vi "ocw.vi"(1 "in":string) -> ()   [LabVIEW 2010]
doc: "OCW v3.0\n\nCopyright 2008 by Will Grover\n\nhttp://wgrover.com\n\nPermission is hereby granted, free of charge, to any person obtaining a copy of this software and associated documentation files (the \"Software\"), to deal in the Software without restriction, including without limitation the rights to use, copy, modify, merge, publish, distribute, sublicense, and/or sell copies of the Software, and to permit persons to whom the Software is furnished to do so, subject to the following conditions:\n\nThe above copyright notice and this permission notice shall be included in all copies or substantial portions of the Software.\n\nTHE SOFTWARE IS PROVIDED \"AS IS\", WITHOUT WARRANTY OF ANY KIND, EXPRESS OR IMPLIED, INCLUDING BUT NOT LIMITED TO THE WARRANTIES OF MERCHANTABILITY, FITNESS FOR A PARTICULAR PURPOSE AND NONINFRINGEMENT. IN NO EVENT SHALL THE AUTHORS OR COPYRIGHT HOLDERS BE LIABLE FOR ANY CLAIM, DAMAGES OR OTHER LIABILITY, WHETHER IN AN ACTION OF CONTRACT, TORT OR OTHERWISE, ARISING FROM, OUT OF OR IN CONNECTION WITH THE SOFTWARE OR THE USE OR OTHER DEALINGS IN THE SOFTWARE."
uses:
  Instance           1 11Saved   ocw .vi
panel:
  out "Subfunction stack":string[](array[string])=["pumpright", "main"]
  in  "Escape":bool
  out "Messages":string
  # "Make sure listener.vi is running before running this VI."
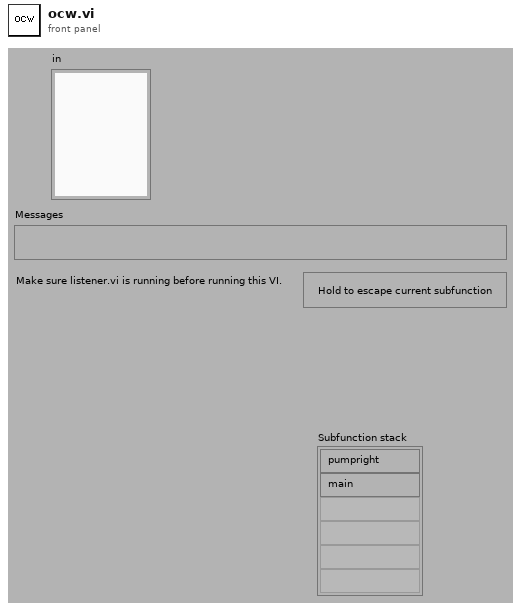
[diagram p1: front panel]
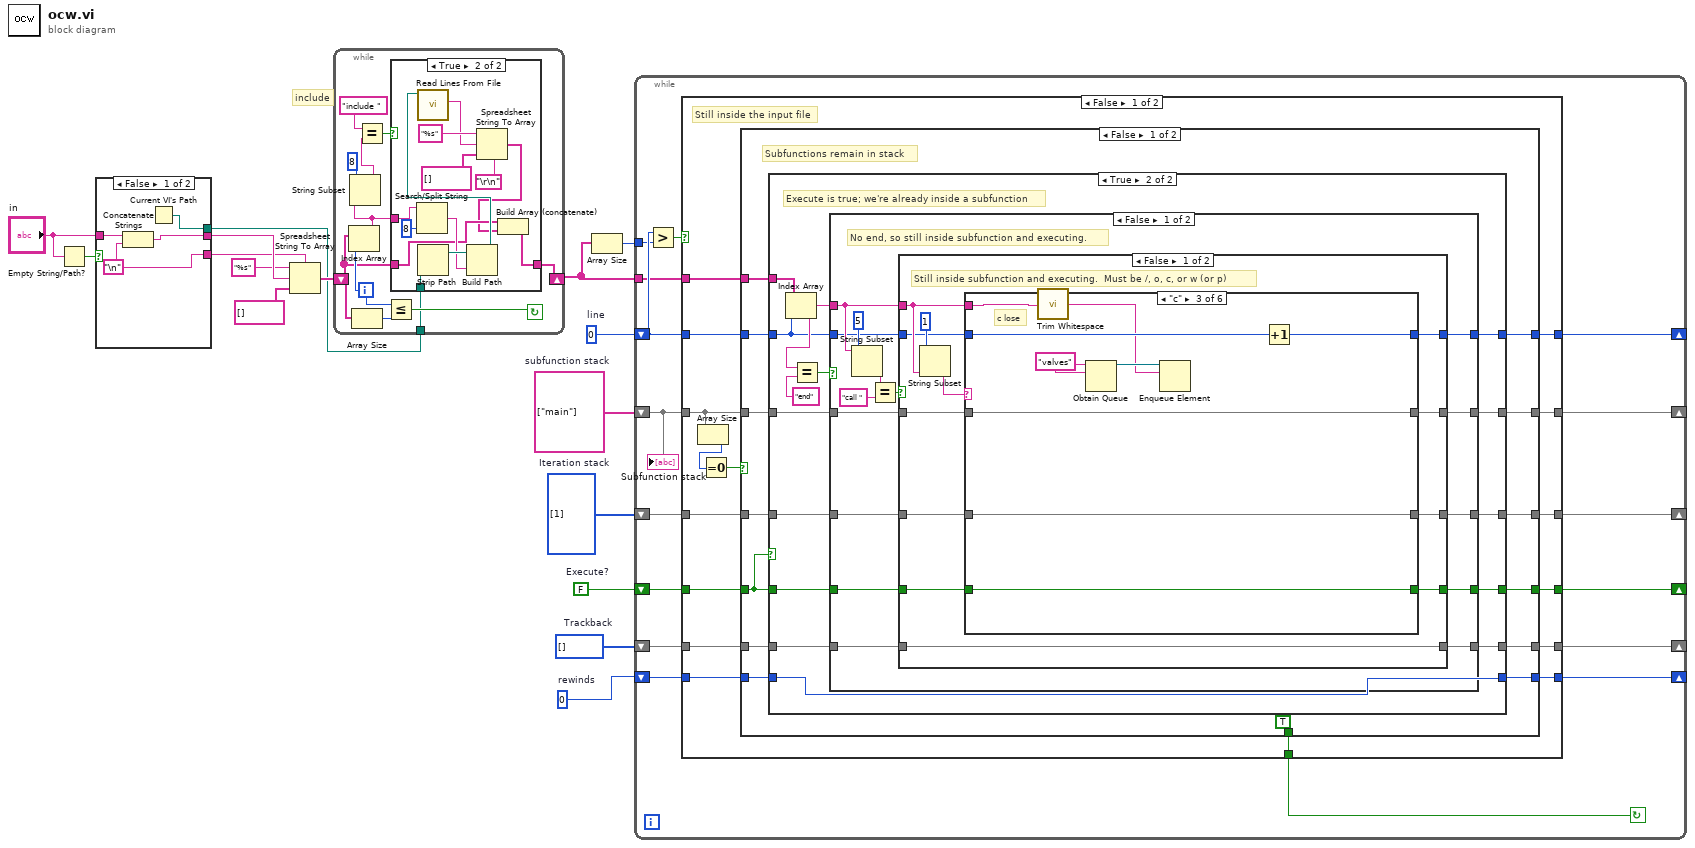
[diagram p0: block diagram]
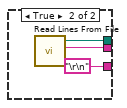
[diagram p2: hidden frame]
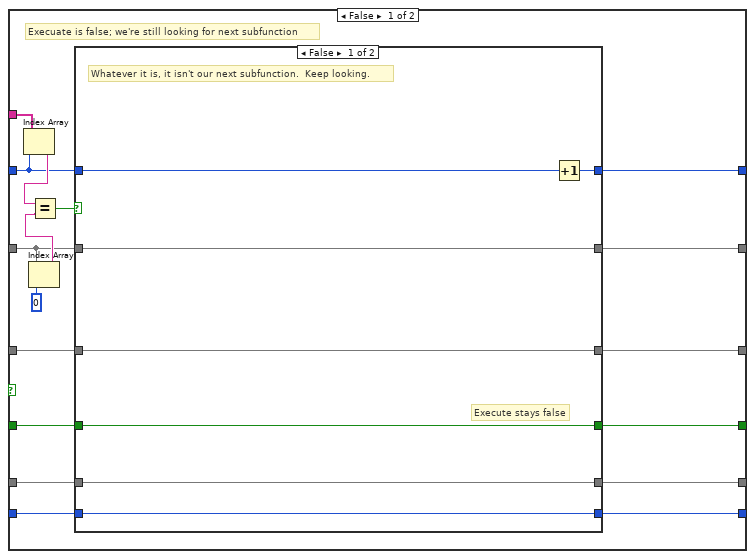
[diagram p4: hidden frame]
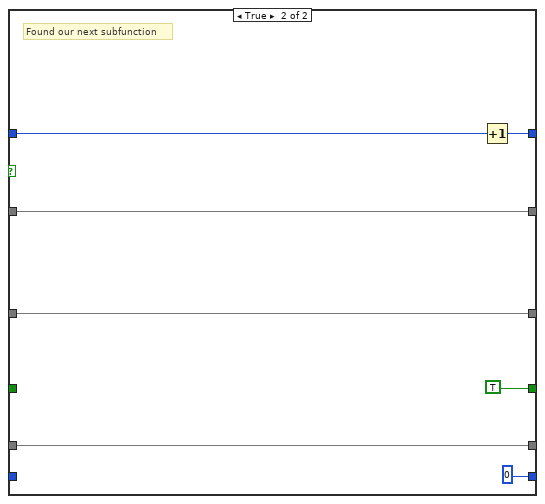
[diagram p5: hidden frame]
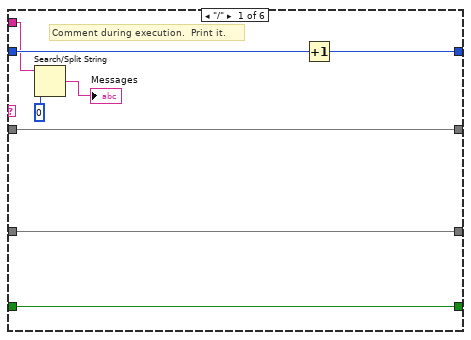
[diagram p6: hidden frame]
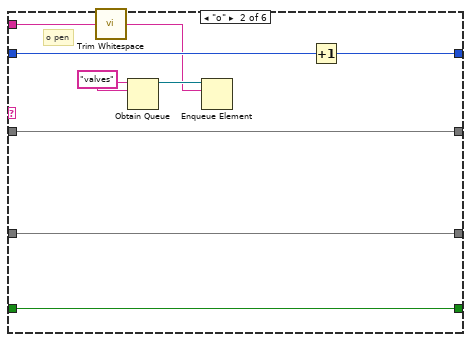
[diagram p7: hidden frame]
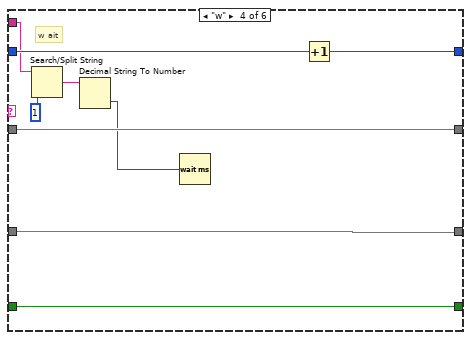
[diagram p8: hidden frame]
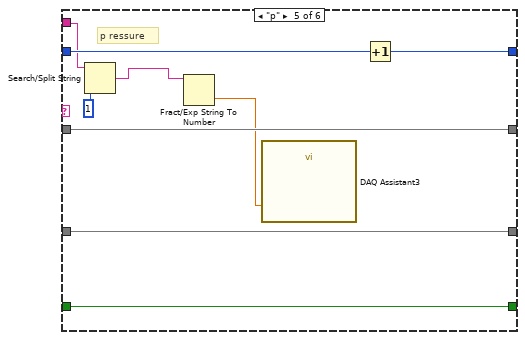
[diagram p9: hidden frame]
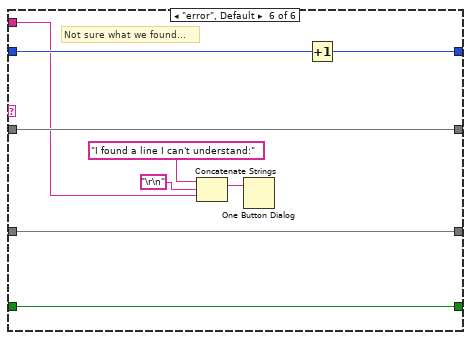
[diagram p10: hidden frame]
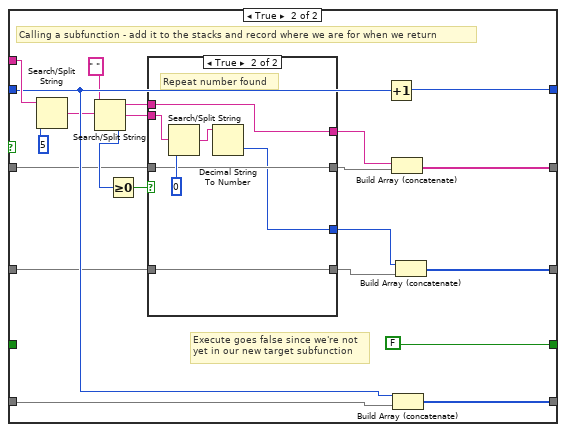
[diagram p11: hidden frame]
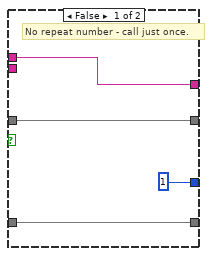
[diagram p12: hidden frame]
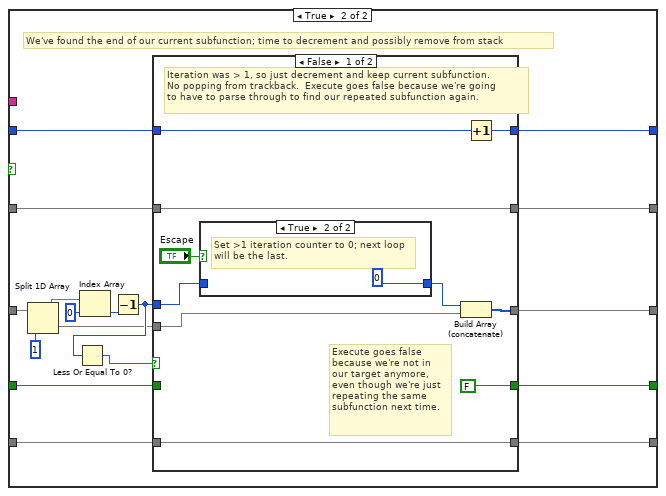
[diagram p13: hidden frame]
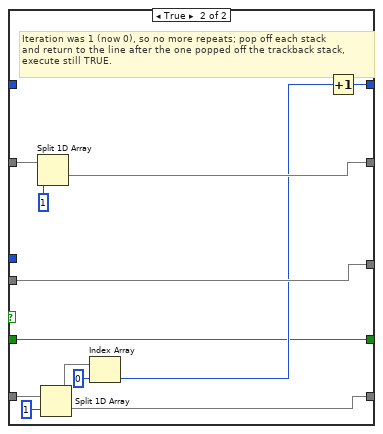
[diagram p15: hidden frame]
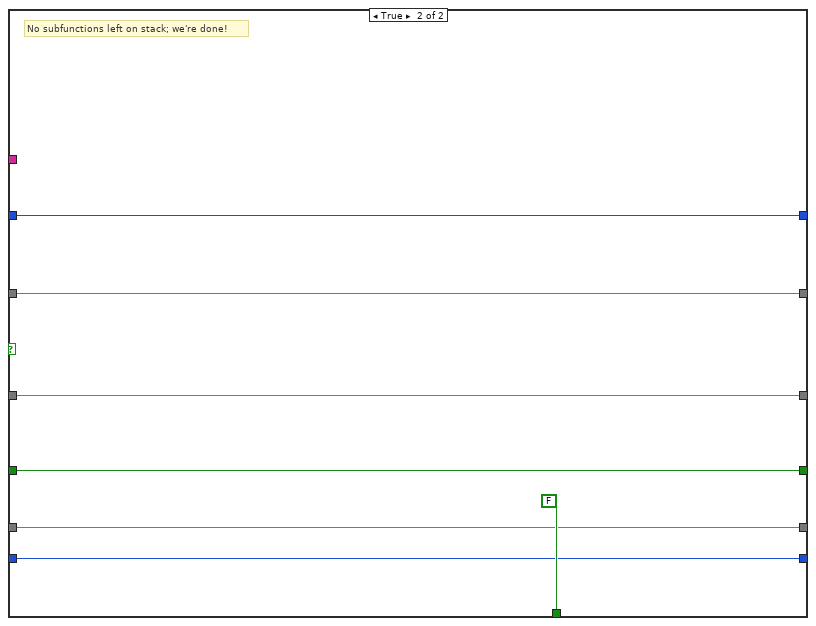
[diagram p16: hidden frame]
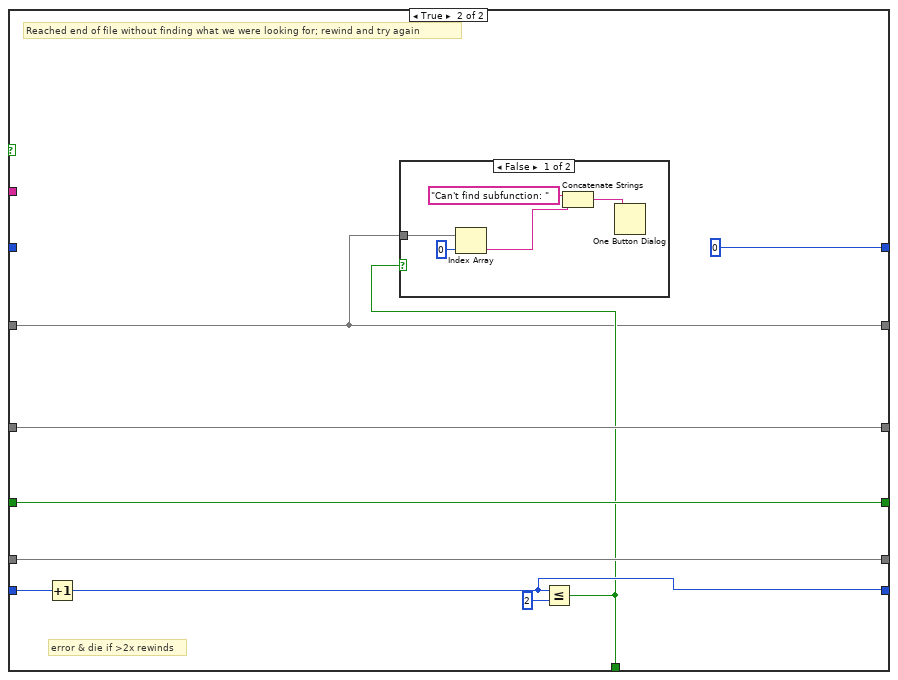
[diagram p17: hidden frame]
diagram:
  w9 = 0  # rewinds
  w11 = i32[] []  # Trackback
  w13 = 0  # line
  w14 = FALSE  # Execute?
  w15 = i32[] [1]  # Iteration stack
  w16 = string[] ["main"]  # subfunction stack
  # "include"
  n1 = Empty String/Path?(string/path="in") -> (empty?=w2:bool)
  n2 = case shown="False" w2 {
    tunnel: [w17 w23] -> w8
    tunnel: [w20 w22] -> w4
    tunnel: "in" -> [w19 _]
    tunnel: [w18 "\r\n"] -> w1
    frame False {
      w18 = "\n"
      n3 = Concatenate Strings(w19, w18) -> (w17:string)
      n4 = Current VI's Path() -> (path=w20:path)
    }
    frame True {
      n5 = call <vilib>:"Read Lines From File.vi"() -> ("new file path (Not A Path if cancelled)"=w22:path, "line string"=w23:string)  [unwired: 2 in, 6 out]
    }
  }
  n6 = Spreadsheet String To Array(delimiter (Tab)=w1, format string="%s", spreadsheet string=w8, array type (2D Dbl)=string[] [] ("Array Constant")) -> (array=w5:string[])
  n7 = while {
    tunnel: w4 -> [w24]
    shift-left: w5 -> [w26]
    shift-right: [w25] -> w10
    i -> [w34]
    stop <- w32 continue-if-true
    n8 = Index Array(array=w26, index=w34) -> (element=w27:string)
    n9 = String Subset(string=w27, length (rest)=8 ("length")) -> (substring=w30:string)  [unwired: 1 out]
    n10 = Array Size(array=w26) -> (size(s)=w33:i32)
    n11 = Equal?(x="include ", y=w30) -> (x = y?=w28:bool)
    n12 = Less Or Equal?(x=w34, y=w33) -> (x <= y?=w32:bool)
    n13 = case shown="True" w28 {
      tunnel: w27 -> [_ w47]
      tunnel: w26 -> [w35 w38]
      tunnel: [w35 w36] -> w25
      tunnel: w24 -> [_ w46]
      frame False {
      }
      frame True {
        n14 = Search/Split String(string=w47, offset (0)=8) -> (match + rest of string=w44:string)  [unwired: 3 out]
        n15 = Strip Path(path=w46) -> (stripped path=w45:path)  [unwired: 1 out]
        n16 = Build Path(base path=w45, name or relative path=w44) -> (appended path=w39:path)
        n17 = call <vilib>:"Read Lines From File.vi"("file path (dialog if empty)"=w39) -> ("line string"=w40:string)  [unwired: 1 in, 7 out]
        n18 = Spreadsheet String To Array(delimiter (Tab)="\r\n", format string="%s", spreadsheet string=w40, array type (2D Dbl)=string[] [] ("Array Constant")) -> (array=w37:string[])
        n19 = Build Array (concatenate)(w38, w37) -> (w36:string[])
      }
    }
  }
  n20 = Array Size(array=w10) -> (size(s)=w12:i32)
  n21 = while {
    shift-left: w9 -> [w50]
    shift-right: [w49] -> _
    shift-left: w11 -> [w52]
    shift-right: [w51] -> _
    tunnel: w12 -> [w63]
    shift-left: w13 -> [w64]
    shift-right: [w53] -> _
    shift-left: w14 -> [w57]
    shift-right: [w56] -> _
    shift-left: w15 -> [w59]
    shift-right: [w55] -> _
    shift-left: w16 -> [w60]
    shift-right: [w54] -> _
    tunnel: w10 -> [w58]
    stop <- w61 continue-if-true
    n22 = Greater?(x=w64, y=w63) -> (0:w62:bool)
    n23 = case shown="False" w62 {
      tunnel: [w78 w302] -> w61
      tunnel: w60 -> [w75 w301]
      tunnel: w59 -> [w76 w308]
      tunnel: w58 -> [w77 _]
      tunnel: w57 -> [w74 w307]
      tunnel: w64 -> [w73 _]
      tunnel: [w72 w307] -> w56
      tunnel: [w71 w308] -> w55
      tunnel: [w70 w301] -> w54
      tunnel: [w69 0] -> w53
      tunnel: w52 -> [w68 w306]
      tunnel: [w67 w306] -> w51
      tunnel: w50 -> [w66 w305]
      tunnel: [w65 w303] -> w49
      frame False {
        # "Still inside the input file"
        n24 = Array Size(array=w75) -> (size(s)=w80:i32)
        n25 = Equal To 0?(x=w80) -> (x = 0?=w79:bool)
        n26 = case shown="False" w79 {
          tunnel: [TRUE FALSE] -> w78
          tunnel: w77 -> [w90 _]
          tunnel: w76 -> [w93 w297]
          tunnel: w75 -> [w92 w298]
          tunnel: w74 -> [w94 w296]
          tunnel: w73 -> [w91 w299]
          tunnel: [w89 w296] -> w72
          tunnel: [w88 w297] -> w71
          tunnel: [w87 w298] -> w70
          tunnel: [w86 w299] -> w69
          tunnel: w68 -> [w84 w295]
          tunnel: [w83 w295] -> w67
          tunnel: w66 -> [w82 w294]
          tunnel: [w81 w294] -> w65
          frame False {
            # "Subfunctions remain in stack"
            n27 = case shown="True" w94 {
              tunnel: w94 -> [w107 w134]
              tunnel: w93 -> [w105 w133]
              tunnel: w92 -> [w99 w135]
              tunnel: w91 -> [w100 w136]
              tunnel: w90 -> [w101 w139]
              tunnel: [w106 w132] -> w89
              tunnel: [w104 w131] -> w88
              tunnel: [w103 w130] -> w87
              tunnel: [w102 w129] -> w86
              tunnel: w84 -> [w98 w128]
              tunnel: [w97 w127] -> w83
              tunnel: w82 -> [w96 w126]
              tunnel: [w95 w126] -> w81
              frame False {
                # "Execuate is false; we're still looking for next subfunction"
                n28 = Index Array(array=w101, index=w100) -> (element=w109:string)
                n29 = Index Array(array=w99, index=0 ("Index")) -> (element=w110:string)
                n30 = Equal?(x=w109, y=w110) -> (x = y?=w108:bool)
                n31 = case shown="False" w108 {
                  tunnel: w107 -> [w118 _]
                  tunnel: [w118 TRUE] -> w106
                  tunnel: w105 -> [w117 w122]
                  tunnel: [w117 w122] -> w104
                  tunnel: [w116 w121] -> w103
                  tunnel: [w115 w124] -> w102
                  tunnel: w100 -> [w114 w123]
                  tunnel: w99 -> [w116 w121]
                  tunnel: w98 -> [w113 w120]
                  tunnel: [w113 w120] -> w97
                  tunnel: w96 -> [w112 _]
                  tunnel: [w112 0] -> w95
                  frame False {
                    # "Execute stays false"
                    # "Whatever it is, it isn't our next subfunction.  Keep looking."
                    n32 = Increment(x=w114) -> (x+1=w115:i32)
                  }
                  frame True {
                    # "Found our next subfunction"
                    n33 = Increment(x=w123) -> (x+1=w124:i32)
                  }
                }
              }
              frame True {
                # "Execute is true; we're already inside a subfunction"
                n34 = Index Array(array=w139, index=w136) -> (element=w140:string)
                n35 = Equal?(x=w140, y="end") -> (x = y?=w137:bool)
                n36 = case shown="False" w137 {
                  tunnel: w136 -> [w147 w256]
                  tunnel: w135 -> [w150 w257]
                  tunnel: w134 -> [w148 w262]
                  tunnel: w133 -> [w149 w269]
                  tunnel: [w143 w261] -> w132
                  tunnel: [w146 w260] -> w131
                  tunnel: [w145 w259] -> w130
                  tunnel: [w144 w258] -> w129
                  tunnel: w140 -> [w151 _]
                  tunnel: w128 -> [w142 w255]
                  tunnel: [w141 w254] -> w127
                  frame False {
                    # "No end, so still inside subfunction and executing."
                    n37 = String Subset(string=w151, length (rest)=5 ("length")) -> (substring=w154:string)  [unwired: 1 out]
                    n38 = Equal?(x=w154, y="call ") -> (x = y?=w152:bool)
                    n39 = case shown="False" w152 {
                      tunnel: w151 -> [w165 w237]
                      tunnel: w150 -> [w163 w223]
                      tunnel: w149 -> [w162 w225]
                      tunnel: w148 -> [w161 _]
                      tunnel: w147 -> [w157 w233]
                      tunnel: [w159 w241] -> w146
                      tunnel: [w158 w240] -> w145
                      tunnel: [w164 w239] -> w144
                      tunnel: [w160 FALSE] -> w143
                      tunnel: w142 -> [w156 w234]
                      tunnel: [w156 w235] -> w141
                      frame False {
                        # "Still inside subfunction and executing.  Must be /, o, c, or w (or p)"
                        n40 = String Subset(string=w165, length (rest)=1 ("length")) -> (substring=w166:string)  [unwired: 1 out]
                        n41 = case shown="\"c\"" w166 {
                          tunnel: w165 -> [w170 w179 w188 w195 w206 w213]
                          tunnel: [w175 w184 w193 w202 w211 w219] -> w164
                          tunnel: w163 -> [w173 w182 w191 w200 w209 w220]
                          tunnel: w162 -> [w172 w181 w190 w199 w208 w217]
                          tunnel: w161 -> [w171 w180 w189 w198 w207 w216]
                          tunnel: [w171 w180 w189 w198 w207 w216] -> w160
                          tunnel: [w172 w181 w190 w199 w208 w217] -> w159
                          tunnel: [w173 w182 w191 w200 w209 w220] -> w158
                          tunnel: w157 -> [w174 w183 w192 w201 w210 w218]
                          frame "/" {
                            # "Comment during execution.  Print it."
                            n42 = Search/Split String(string=w170, offset (0)=0) -> (match + rest of string=→"Messages":string)  [unwired: 3 out]
                            n43 = Increment(x=w174) -> (x+1=w175:i32)
                          }
                          frame "o" {
                            w178 = "valves" ("name (unnamed)")
                            # "o pen"
                            n44 = call <vilib>:"Trim Whitespace.vi"("string"=w179) -> ("trimmed string"=w176:string)  [unwired: 1 in]
                            n45 = Obtain Queue(name (unnamed)=w178, element data type=w178) -> (queue out=w177:refnum<queue>)  [unwired: 3 in, 2 out]
                            n46 = Enqueue Element(queue=w177, element=w176) -> ()  [unwired: 1 in, 4 out]
                            n47 = Increment(x=w183) -> (x+1=w184:i32)
                          }
                          frame "c" {
                            w187 = "valves" ("name (unnamed)")
                            # "c lose"
                            n48 = call <vilib>:"Trim Whitespace.vi"("string"=w188) -> ("trimmed string"=w185:string)  [unwired: 1 in]
                            n49 = Obtain Queue(name (unnamed)=w187, element data type=w187) -> (queue out=w186:refnum<queue>)  [unwired: 3 in, 2 out]
                            n50 = Enqueue Element(queue=w186, element=w185) -> ()  [unwired: 1 in, 4 out]
                            n51 = Increment(x=w192) -> (x+1=w193:i32)
                          }
                          frame "w" {
                            # "w ait"
                            n52 = Search/Split String(string=w195, offset (0)=1) -> (match + rest of string=w197:string)  [unwired: 3 out]
                            n53 = Decimal String To Number(string=w197) -> (number=w194:i32)  [unwired: 3 out]
                            n54 = Wait (ms)(milliseconds to wait=w194) -> ()  [unwired: 1 out]
                            n55 = Increment(x=w201) -> (x+1=w202:i32)
                          }
                          frame "p" {
                            # "p ressure"
                            n56 = Search/Split String(string=w206, offset (0)=1) -> (match + rest of string=w204:string)  [unwired: 3 out]
                            n57 = Fract/Exp String To Number(string=w204) -> (number=w203:dbl)  [unwired: 4 out]
                            n58 = call "DAQ Assistant3"("data"=w203) -> ()  [unwired: 3 in, 8 out]
                            n59 = Increment(x=w210) -> (x+1=w211:i32)
                          }
                          frame "error", Default {
                            # "Not sure what we found..."
                            n60 = Concatenate Strings("I found a line I can't understand:" ("message"), "\r\n", w213) -> (w212:string)
                            n61 = One Button Dialog(message=w212) -> ()  [unwired: 2 out]
                            n62 = Increment(x=w218) -> (x+1=w219:i32)
                          }
                        }
                      }
                      frame True {
                        # "Execute goes false since we're not\nyet in our new target subfunction"
                        # "Calling a subfunction - add it to the stacks and record where we are for when we return"
                        n63 = Search/Split String(string=w237, offset (0)=5) -> (match + rest of string=w232:string)  [unwired: 3 out]
                        n64 = Search/Split String(string=w232, search string/char (-)=" ") -> (substring before match=w228:string, match + rest of string=w227:string, offset of match=w230:i32)  [unwired: 1 out]
                        n65 = Greater Or Equal To 0?(x=w230) -> (x >= 0?=w229:bool)
                        n66 = case shown="True" w229 {
                          tunnel: w228 -> [w245 w250]
                          tunnel: w227 -> [_ w251]
                          tunnel: [w245 w250] -> w226
                          tunnel: w225 -> [w244 w249]
                          tunnel: [w244 w249] -> w224
                          tunnel: w223 -> [w243 w248]
                          tunnel: [w243 w248] -> w222
                          tunnel: [1 ("Input Element") w246] -> w221
                          frame False {
                            # "No repeat number - call just once."
                          }
                          frame True {
                            # "Repeat number found"
                            n67 = Search/Split String(string=w251, offset (0)=0) -> (match + rest of string=w247:string)  [unwired: 3 out]
                            n68 = Decimal String To Number(string=w247) -> (number=w246:i32)  [unwired: 3 out]
                          }
                        }
                        n69 = Increment(x=w233) -> (x+1=w239:i32)
                        n70 = Build Array (concatenate)(w226, w222) -> (w240:string[])
                        n71 = Build Array (concatenate)(w233, w234) -> (w235:i32[])
                        n72 = Build Array (concatenate)(w221, w224) -> (w241:i32[])
                      }
                    }
                  }
                  frame True {
                    # "We've found the end of our current subfunction; time to decrement and possibly remove from stack"
                    n73 = Split 1D Array(array=w269, index=1) -> (first subarray=w267:i32[], second subarray=w263:i32[])
                    n74 = Index Array(array=w267, index=0 ("Index")) -> (element=w265:i32)
                    n75 = Decrement(x=w265) -> (x-1=w264:i32)
                    n76 = Less Or Equal To 0?(x=w264) -> (x <= 0?=w253:bool)
                    n77 = case shown="False" w253 {
                      tunnel: w264 -> [w272 _]
                      tunnel: w263 -> [w279 w293]
                      tunnel: w262 -> [_ w282]
                      tunnel: [FALSE w282] -> w261
                      tunnel: [w277 w293] -> w260
                      tunnel: [w274 w290] -> w259
                      tunnel: [w276 w289] -> w258
                      tunnel: w257 -> [w274 w291]
                      tunnel: w256 -> [w275 _]
                      tunnel: w255 -> [w273 w287]
                      tunnel: [w273 w286] -> w254
                      frame False {
                        # "Execute goes false\nbecause we're not in\nour target anymore,\neven though we're just\nrepeating the same\nsubfunction next time."
                        # "Iteration was > 1, so just decrement and keep current subfunction.\nNo popping from trackback.  Execute goes false because we're going\nto have to parse through to find our repeated subfunction again."
                        n78 = case shown="True" "Escape" {
                          tunnel: w272 -> [w280 _]
                          tunnel: [w280 0] -> w271
                          frame False {
                          }
                          frame True {
                            # "Set >1 iteration counter to 0; next loop\nwill be the last."
                          }
                        }
                        n79 = Build Array (concatenate)(w271, w279) -> (w277:i32[])
                        n80 = Increment(x=w275) -> (x+1=w276:i32)
                      }
                      frame True {
                        # "Iteration was 1 (now 0), so no more repeats; pop off each stack\nand return to the line after the one popped off the trackback stack, \nexecute still TRUE."
                        n81 = Split 1D Array(array=w291, index=1) -> (second subarray=w290:string[])  [unwired: 1 out]
                        n82 = Split 1D Array(array=w287, index=1) -> (first subarray=w285:i32[], second subarray=w286:i32[])
                        n83 = Index Array(array=w285, index=0 ("Index")) -> (element=w283:i32)
                        n84 = Increment(x=w283) -> (x+1=w289:i32)
                      }
                    }
                  }
                }
              }
            }
          }
          frame True {
            # "No subfunctions left on stack; we're done!"
          }
        }
      }
      frame True {
        # "error & die if >2x rewinds"
        # "Reached end of file without finding what we were looking for; rewind and try again"
        n85 = Increment(x=w305) -> (x+1=w303:i32)
        n86 = Less Or Equal?(x=w303, y=2) -> (x <= y?=w302:bool)
        n87 = case shown="False" w302 {
          tunnel: w301 -> [w313 _]
          frame False {
            n88 = Index Array(array=w313, index=0 ("Index")) -> (element=w311:string)
            n89 = Concatenate Strings("Can't find subfunction: " ("Substring"), w311) -> (w310:string)
            n90 = One Button Dialog(message=w310) -> ()  [unwired: 2 out]
          }
          frame True {
            # "do nothing"
          }
        }
      }
    }
    "Subfunction stack" <- w60
  }
